vi "Lab Panel V5.29.vi"() -> ()   [LabVIEW 2013] (continued)
                            n1772 = local write "mail control"("END") -> ()
                            n1773 = Bundle(cluster=w3324) -> (w3325:T4)  [unwired: 3 in]
                            n1774 = local write "RUN LAB05-2"(w3322) -> ()
                            n1775 = local write "O/I  LAB05-2"(w3322) -> ()
                            n1776 = local write "run lab05-2"(w3322) -> ()
                            n1777 = local write "DISP LAB05-2"(w3325) -> ()
                          }
                          frame #1 {
                            n1778 = TDMS Close(11:w3326) -> (0:w3327:errorcluster)  [unwired: 1 in, 1 out]
                            n1779 = local write "data file error"(w3327) -> ()
                          }
                          frame #2 {
                            n1780 = stacked-sequence {
                              tunnel: "LAB05-2" -> [w3335 w3341]
                              tunnel: w3332 -> [_ w3340]
                              tunnel: w3331 -> [_ w3339]
                              tunnel: w3330 -> [_ w3338]
                              tunnel: w3329 -> [_ w3337]
                              tunnel: w3328 -> [_ w3336]
                              frame #0 {
                                n1781 = call "sub vi - defrag tdms v1.vi"("panel id"=w3335) -> ("error out"=w3334:errorcluster)  [unwired: 10 in]
                                n1782 = local write "data file error"(w3334) -> ()
                              }
                              frame #1 {
                                n1783 = Bundle("STATUS"=w3340, "OUT SERVER ADDRESS"=w3339, "FROM ACCOUNT"=w3338, "Mail Test File To:"=w3337, "Mail Test Fail"=w3336) -> (w3343:T26)  [unwired: 1 in]
                                n1784 = call "Save data file (pass-fail) v5.vi"("Input Cluster"=w3343, "panel id"=w3341) -> ("network file save error"=w3342:errorcluster)  [unwired: 8 in, 1 out]
                                n1785 = local write "data file error"(w3342) -> ()
                              }
                            }
                          }
                        }
                      }
                    }
                  }
                }
              }
            }
            n1786 = global write "Global display 2.vi" "Mail test file to:"(w2851) -> ()
            n1787 = local read "Network Directory"() -> (w2857:path)
            n1788 = global write "Global 1.vi" "Network Drive"(w2857) -> ()
          }
          frame #8 {
            # "disable functions"
            n1789 = stacked-sequence {
              tunnel: w3353 -> [w3367 _ w3424]
              tunnel: w3352 -> [w3362 _ w3423]
              tunnel: w3351 -> [w3361 _ w3422]
              tunnel: w3350 -> [w3359 _ w3421]
              tunnel: w3349 -> [w3360 _ w3420]
              tunnel: w3348 -> [_ w3384 w3419]
              tunnel: w3347 -> [_ w3385 w3418]
              tunnel: w3346 -> [_ w3386 w3417]
              tunnel: w3345 -> [_ w3387 w3416]
              tunnel: w3344 -> [_ w3388 w3415]
              frame #0 {
                n1790 = Select(t=2, s=w3359, f=0) -> (s? t:f=w3355:i32)
                n1791 = Select(t=2, s=w3361, f=0) -> (s? t:f=w3356:i32)
                n1792 = Select(t=2, s=w3360, f=0) -> (s? t:f=w3354:i32)
                n1793 = Select(t=2, s=w3367, f=0) -> (s? t:f=w3358:i32)
                n1794 = Select(t=2, s=w3362, f=0) -> (s? t:f=w3357:i32)
                n1795 = property on="SELECT LAB02-2" class="RadioBtnsControl (strict)"("DisabledEnum"=w3355) -> ()  [unwired: 2 in, 2 out]
                n1796 = property on="SELECT LAB02-1" class="RadioBtnsControl (strict)"("DisabledEnum"=w3356) -> ()  [unwired: 2 in, 2 out]
                n1797 = property on="SELECT LAB03-1" class="RadioBtnsControl (strict)"("DisabledEnum"=w3354) -> ()  [unwired: 2 in, 2 out]
                n1798 = property on="SELECT LAB01-1" class="RadioBtnsControl (strict)"("DisabledEnum"=w3358) -> ()  [unwired: 2 in, 2 out]
                n1799 = property on="SELECT LAB01-2" class="RadioBtnsControl (strict)"("DisabledEnum"=w3357) -> ()  [unwired: 2 in, 2 out]
                n1800 = Not(x=w3367) -> (.not. x?=w3368:bool)
                n1801 = property on="RESULT LAB01-1" class="Bool (strict)"("Visible"=w3368) -> ()  [unwired: 2 in, 2 out]
                n1802 = Not(x=w3362) -> (.not. x?=w3366:bool)
                n1803 = Not(x=w3361) -> (.not. x?=w3365:bool)
                n1804 = Not(x=w3359) -> (.not. x?=w3364:bool)
                n1805 = property on="RESULT LAB01-2" class="Bool (strict)"("Visible"=w3366) -> ()  [unwired: 2 in, 2 out]
                n1806 = Not(x=w3360) -> (.not. x?=w3363:bool)
                n1807 = property on="RESULT LAB02-1" class="Bool (strict)"("Visible"=w3365) -> ()  [unwired: 2 in, 2 out]
                n1808 = property on="RESULT LAB02-2" class="Bool (strict)"("Visible"=w3364) -> ()  [unwired: 2 in, 2 out]
                n1809 = property on="RESULT LAB03-1" class="Bool (strict)"("Visible"=w3363) -> ()  [unwired: 2 in, 2 out]
                n1810 = property on="SET LAB01-1" class="Clust (strict)"("DisabledEnum"=w3358) -> ()  [unwired: 2 in, 2 out]
                n1811 = property on="SET LAB01-2" class="Clust (strict)"("DisabledEnum"=w3357) -> ()  [unwired: 2 in, 2 out]
                n1812 = property on="SET LAB02-1" class="Clust (strict)"("DisabledEnum"=w3356) -> ()  [unwired: 2 in, 2 out]
                n1813 = property on="SET LAB02-2" class="Clust (strict)"("DisabledEnum"=w3355) -> ()  [unwired: 2 in, 2 out]
                n1814 = property on="SET LAB03-1" class="Clust (strict)"("DisabledEnum"=w3354) -> ()  [unwired: 2 in, 2 out]
                n1815 = property on="O/I  LAB01-1" class="Bool (strict)"("DisabledEnum"=w3358) -> ()  [unwired: 2 in, 2 out]
                n1816 = property on="O/I  LAB01-2" class="Bool (strict)"("DisabledEnum"=w3357) -> ()  [unwired: 2 in, 2 out]
                n1817 = property on="O/I  LAB02-1" class="Bool (strict)"("DisabledEnum"=w3356) -> ()  [unwired: 2 in, 2 out]
                n1818 = property on="O/I  LAB02-2" class="Bool (strict)"("DisabledEnum"=w3355) -> ()  [unwired: 2 in, 2 out]
                n1819 = property on="O/I  LAB03-1" class="Bool (strict)"("DisabledEnum"=w3354) -> ()  [unwired: 2 in, 2 out]
              }
              frame #1 {
                n1820 = Select(t=2, s=w3388, f=0) -> (s? t:f=w3379:i32)
                n1821 = Select(t=2, s=w3387, f=0) -> (s? t:f=w3380:i32)
                n1822 = Select(t=2, s=w3384, f=0) -> (s? t:f=w3383:i32)
                n1823 = Select(t=2, s=w3385, f=0) -> (s? t:f=w3382:i32)
                n1824 = Select(t=2, s=w3386, f=0) -> (s? t:f=w3381:i32)
                n1825 = property on="SELECT LAB05-2" class="RadioBtnsControl (strict)"("DisabledEnum"=w3379) -> ()  [unwired: 2 in, 2 out]
                n1826 = property on="SELECT LAB05-1" class="RadioBtnsControl (strict)"("DisabledEnum"=w3380) -> ()  [unwired: 2 in, 2 out]
                n1827 = property on="SELECT LAB03-2" class="RadioBtnsControl (strict)"("DisabledEnum"=w3383) -> ()  [unwired: 2 in, 2 out]
                n1828 = property on="SELECT LAB04-1" class="RadioBtnsControl (strict)"("DisabledEnum"=w3382) -> ()  [unwired: 2 in, 2 out]
                n1829 = property on="SELECT LAB04-2" class="RadioBtnsControl (strict)"("DisabledEnum"=w3381) -> ()  [unwired: 2 in, 2 out]
                n1830 = property on="SET LAB05-2" class="Clust (strict)"("DisabledEnum"=w3379) -> ()  [unwired: 2 in, 2 out]
                n1831 = property on="SET LAB05-1" class="Clust (strict)"("DisabledEnum"=w3380) -> ()  [unwired: 2 in, 2 out]
                n1832 = property on="SET LAB03-2" class="Clust (strict)"("DisabledEnum"=w3383) -> ()  [unwired: 2 in, 2 out]
                n1833 = property on="SET LAB04-1" class="Clust (strict)"("DisabledEnum"=w3382) -> ()  [unwired: 2 in, 2 out]
                n1834 = property on="SET LAB04-2" class="Clust (strict)"("DisabledEnum"=w3381) -> ()  [unwired: 2 in, 2 out]
                n1835 = property on="O/I  LAB05-2" class="Bool (strict)"("DisabledEnum"=w3379) -> ()  [unwired: 2 in, 2 out]
                n1836 = property on="O/I  LAB05-1" class="Bool (strict)"("DisabledEnum"=w3380) -> ()  [unwired: 2 in, 2 out]
                n1837 = property on="O/I  LAB04-1" class="Bool (strict)"("DisabledEnum"=w3382) -> ()  [unwired: 2 in, 2 out]
                n1838 = property on="O/I  LAB04-2" class="Bool (strict)"("DisabledEnum"=w3381) -> ()  [unwired: 2 in, 2 out]
                n1839 = property on="O/I  LAB03-2" class="Bool (strict)"("DisabledEnum"=w3383) -> ()  [unwired: 2 in, 2 out]
                n1840 = Not(x=w3388) -> (.not. x?=w3389:bool)
                n1841 = Not(x=w3387) -> (.not. x?=w3390:bool)
                n1842 = Not(x=w3386) -> (.not. x?=w3391:bool)
                n1843 = property on="RESULT LAB05-2" class="Bool (strict)"("Visible"=w3389) -> ()  [unwired: 2 in, 2 out]
                n1844 = property on="RESULT LAB05-1" class="Bool (strict)"("Visible"=w3390) -> ()  [unwired: 2 in, 2 out]
                n1845 = Not(x=w3385) -> (.not. x?=w3392:bool)
                n1846 = property on="RESULT LAB04-2" class="Bool (strict)"("Visible"=w3391) -> ()  [unwired: 2 in, 2 out]
                n1847 = Not(x=w3384) -> (.not. x?=w3393:bool)
                n1848 = property on="RESULT LAB04-1" class="Bool (strict)"("Visible"=w3392) -> ()  [unwired: 2 in, 2 out]
                n1849 = property on="RESULT LAB03-2" class="Bool (strict)"("Visible"=w3393) -> ()  [unwired: 2 in, 2 out]
              }
              frame #2 {
                # "disable calibrate if any test running"
                n1850 = Or(x=w3416, y=w3415) -> (x .or. y?=w3409:bool)
                n1851 = Or(x=w3418, y=w3417) -> (x .or. y?=w3411:bool)
                n1852 = Or(x=w3422, y=w3421) -> (x .or. y?=w3413:bool)
                n1853 = Or(x=w3420, y=w3419) -> (x .or. y?=w3412:bool)
                n1854 = Or(x=w3424, y=w3423) -> (x .or. y?=w3414:bool)
                n1855 = Or(x=w3412, y=w3411) -> (x .or. y?=w3410:bool)
                n1856 = Or(x=w3414, y=w3413) -> (x .or. y?=w3408:bool)
                n1857 = Or(x=w3410, y=w3409) -> (x .or. y?=w3407:bool)
                n1858 = Or(x=w3408, y=w3407) -> (x .or. y?=w3404:bool)
                "Any Test Running" <- w3404
                n1859 = case shown="False" w3404 {
                  tunnel: [0 2] -> w3406
                  frame False {
                  }
                  frame True {
                  }
                }
                n1860 = property on="JIG TEST" class="Clust (strict)"("DisabledEnum"=w3406) -> ()  [unwired: 2 in, 2 out]
                n1861 = property on="Network Directory" class="Path"("DisabledEnum"=w3406) -> ()  [unwired: 2 in, 2 out]
                n1862 = property on="MAIL SETTINGS" class="Clust (strict)"("DisabledEnum"=w3406) -> ()  [unwired: 2 in, 2 out]
                n1863 = property on="SET (cal)" class="Bool (strict)"("DisabledEnum"=w3406) -> ()  [unwired: 2 in, 2 out]
                n1864 = property on="ADMIN" class="Bool (strict)"("DisabledEnum"=0) -> ()  [unwired: 2 in, 2 out]
              }
            }
          }
          frame #9 {
            # "drive jigs"
            n1865 = stacked-sequence {
              frame #0 {
                # "jig on"
                n1866 = local read "jig cycle"() -> (w3432:dbl)
                n1867 = property on="JIG TEST" class="Clust (strict)"() -> ("DisabledEnum"=w3429:T16)  [unwired: 2 in, 2 out]
                n1868 = Equal?(x=w3429, y=2) -> (x = y?=w3428:bool)
                n1869 = Equal?(x=w3432, y=0) -> (x = y?=w3430:bool)
                n1870 = And(x=w3430, y=w3428) -> (x .and. y?=w3427:bool)
                n1871 = case shown="True" w3427 {
                  frame False {
                  }
                  frame True {
                    n1872 = local read "run lab01-1"() -> (w3443:bool)
                    n1873 = local read "run lab01-2"() -> (w3442:bool)
                    n1874 = local read "run lab02-1"() -> (w3441:bool)
                    n1875 = local read "run lab02-2"() -> (w3440:bool)
                    n1876 = local read "run lab03-1"() -> (w3439:bool)
                    n1877 = local read "run lab03-2"() -> (w3438:bool)
                    n1878 = local read "run lab04-1"() -> (w3437:bool)
                    n1879 = local read "run lab04-2"() -> (w3436:bool)
                    n1880 = local read "run lab05-1"() -> (w3435:bool)
                    n1881 = local read "run lab05-2"() -> (w3434:bool)
                    n1882 = local write "JIG LAB03-2"(w3438) -> ()
                    n1883 = local write "JIG LAB01-1"(w3443) -> ()
                    n1884 = local write "JIG LAB01-2"(w3442) -> ()
                    n1885 = local write "JIG LAB02-1"(w3441) -> ()
                    n1886 = local write "JIG LAB02-2"(w3440) -> ()
                    n1887 = local write "JIG LAB03-1"(w3439) -> ()
                    n1888 = local write "JIG LAB04-1"(w3437) -> ()
                    n1889 = local write "JIG LAB04-2"(w3436) -> ()
                    n1890 = local write "JIG LAB05-1"(w3435) -> ()
                    n1891 = local write "JIG LAB05-2"(w3434) -> ()
                  }
                }
              }
              frame #1 {
                # "jig off"
                n1892 = local read "jig cycle"() -> (w3450:dbl)
                n1893 = local read "on loops"() -> (w3449:dbl)
                n1894 = property on="JIG TEST" class="Clust (strict)"() -> ("DisabledEnum"=w3448:T16)  [unwired: 2 in, 2 out]
                n1895 = Equal?(x=w3448, y=2) -> (x = y?=w3446:bool)
                n1896 = Equal?(x=w3450, y=w3449) -> (x = y?=w3445:bool)
                n1897 = And(x=w3445, y=w3446) -> (x .and. y?=w3444:bool)
                n1898 = case shown="True" w3444 {
                  frame False {
                  }
                  frame True {
                    w3501 = FALSE
                    w3502 = TRUE
                    w3500 = 2
                    n1899 = local read "SELECT LAB05-2"() -> (w3491:T3)
                    n1900 = local read "SELECT LAB04-2"() -> (w3493:T3)
                    n1901 = local read "SELECT LAB04-1"() -> (w3494:T3)
                    n1902 = local read "SELECT LAB05-1"() -> (w3492:T3)
                    n1903 = local read "SELECT LAB03-2"() -> (w3495:T3)
                    n1904 = local read "SELECT LAB02-1"() -> (w3498:T3)
                    n1905 = local read "SELECT LAB03-1"() -> (w3496:T3)
                    n1906 = local read "SELECT LAB02-2"() -> (w3497:T3)
                    n1907 = local read "SELECT LAB01-2"() -> (w3499:T3)
                    n1908 = local read "run lab05-1"() -> (w3461:bool)
                    n1909 = local read "run lab05-2"() -> (w3460:bool)
                    n1910 = local read "SELECT LAB01-1"() -> (w3503:T3)
                    n1911 = local read "run lab04-2"() -> (w3462:bool)
                    n1912 = local read "run lab04-1"() -> (w3463:bool)
                    n1913 = local read "run lab01-1"() -> (w3479:bool)
                    n1914 = local read "run lab01-2"() -> (w3468:bool)
                    n1915 = local read "run lab03-2"() -> (w3464:bool)
                    n1916 = local read "run lab03-1"() -> (w3465:bool)
                    n1917 = local read "run lab02-1"() -> (w3467:bool)
                    n1918 = local read "run lab02-2"() -> (w3466:bool)
                    n1919 = Equal?(x=w3500, y=w3496) -> (x = y?=w3474:bool)
                    n1920 = Equal?(x=w3500, y=w3495) -> (x = y?=w3473:bool)
                    n1921 = Equal?(x=w3500, y=w3494) -> (x = y?=w3472:bool)
                    n1922 = Equal?(x=w3500, y=w3493) -> (x = y?=w3471:bool)
                    n1923 = Equal?(x=w3500, y=w3492) -> (x = y?=w3470:bool)
                    n1924 = Equal?(x=w3500, y=w3491) -> (x = y?=w3469:bool)
                    n1925 = Equal?(x=w3500, y=w3503) -> (x = y?=w3480:bool)
                    n1926 = Equal?(x=w3500, y=w3498) -> (x = y?=w3476:bool)
                    n1927 = Equal?(x=w3500, y=w3497) -> (x = y?=w3475:bool)
                    n1928 = Equal?(x=w3500, y=w3499) -> (x = y?=w3477:bool)
                    n1929 = And(x=w3471, y=w3462) -> (x .and. y?=w3453:bool)
                    n1930 = And(x=w3474, y=w3465) -> (x .and. y?=w3456:bool)
                    n1931 = And(x=w3472, y=w3463) -> (x .and. y?=w3454:bool)
                    n1932 = And(x=w3469, y=w3460) -> (x .and. y?=w3451:bool)
                    n1933 = And(x=w3475, y=w3466) -> (x .and. y?=w3457:bool)
                    n1934 = And(x=w3473, y=w3464) -> (x .and. y?=w3455:bool)
                    n1935 = And(x=w3470, y=w3461) -> (x .and. y?=w3452:bool)
                    n1936 = And(x=w3477, y=w3468) -> (x .and. y?=w3459:bool)
                    n1937 = And(x=w3480, y=w3479) -> (x .and. y?=w3478:bool)
                    n1938 = And(x=w3476, y=w3467) -> (x .and. y?=w3458:bool)
                    n1939 = Select(t=w3502, s=w3478, f=w3501) -> (s? t:f=w3481:bool)
                    n1940 = Select(t=w3502, s=w3459, f=w3501) -> (s? t:f=w3482:bool)
                    n1941 = Select(t=w3502, s=w3458, f=w3501) -> (s? t:f=w3483:bool)
                    n1942 = Select(t=w3502, s=w3457, f=w3501) -> (s? t:f=w3484:bool)
                    n1943 = Select(t=w3502, s=w3456, f=w3501) -> (s? t:f=w3485:bool)
                    n1944 = Select(t=w3502, s=w3455, f=w3501) -> (s? t:f=w3486:bool)
                    n1945 = Select(t=w3502, s=w3454, f=w3501) -> (s? t:f=w3487:bool)
                    n1946 = Select(t=w3502, s=w3453, f=w3501) -> (s? t:f=w3488:bool)
                    n1947 = Select(t=w3502, s=w3452, f=w3501) -> (s? t:f=w3489:bool)
                    n1948 = Select(t=w3502, s=w3451, f=w3501) -> (s? t:f=w3490:bool)
                    n1949 = local write "JIG LAB03-2"(w3486) -> ()
                    n1950 = local write "JIG LAB02-1"(w3483) -> ()
                    n1951 = local write "JIG LAB02-2"(w3484) -> ()
                    n1952 = local write "JIG LAB01-2"(w3482) -> ()
                    n1953 = local write "JIG LAB03-1"(w3485) -> ()
                    n1954 = local write "JIG LAB01-1"(w3481) -> ()
                    n1955 = local write "JIG LAB05-2"(w3490) -> ()
                    n1956 = local write "JIG LAB04-1"(w3487) -> ()
                    n1957 = local write "JIG LAB05-1"(w3489) -> ()
                    n1958 = local write "JIG LAB04-2"(w3488) -> ()
                  }
                }
              }
            }
          }
          frame #10 {
            # "enable  jig test output if no test busy"
            n1959 = property on="JIG TEST" class="Clust (strict)"() -> ("DisabledEnum"=w3506:T16)  [unwired: 2 in, 2 out]
            n1960 = Equal?(x=w3506, y=0) -> (x = y?=w3504:bool)
            n1961 = case shown="True" w3504 {
              frame False {
              }
              frame True {
                n1962 = local read "JIG TEST"() -> (w3517:T10)
                n1963 = Unbundle(w3517) -> ("LAB01-1"=w3516:bool, "LAB01-2"=w3515:bool, "LAB02-1"=w3514:bool, "LAB02-2"=w3513:bool, "LAB03-1"=w3512:bool, "LAB03-2"=w3511:bool, "LAB04-1"=w3510:bool, "LAB04-2"=w3509:bool, "LAB05-1"=w3508:bool, "LAB05-2"=w3507:bool)
                n1964 = local write "JIG LAB05-1"(w3508) -> ()
                n1965 = local write "JIG LAB05-2"(w3507) -> ()
                n1966 = local write "JIG LAB04-1"(w3510) -> ()
                n1967 = local write "JIG LAB04-2"(w3509) -> ()
                n1968 = local write "JIG LAB03-2"(w3511) -> ()
                n1969 = local write "JIG LAB01-1"(w3516) -> ()
                n1970 = local write "JIG LAB02-1"(w3514) -> ()
                n1971 = local write "JIG LAB03-1"(w3512) -> ()
                n1972 = local write "JIG LAB01-2"(w3515) -> ()
                n1973 = local write "JIG LAB02-2"(w3513) -> ()
              }
            }
          }
          frame #11 {
            w3518 = FALSE
            # "Drive digital output and reset USB and temperature network if required."
            n1974 = global read "Global display 3.vi" "cycle O/F"() -> (w3527:bool)
            n1975 = local read "O/I  LAB05-2"() -> (w3520:bool)
            n1976 = local read "O/I  LAB05-1"() -> (w3522:bool)
            n1977 = local read "JIG LAB05-2"() -> (w3519:bool)
            n1978 = local read "O/I  LAB04-2"() -> (w3524:bool)
            n1979 = local read "JIG LAB05-1"() -> (w3521:bool)
            n1980 = local read "JIG LAB04-2"() -> (w3523:bool)
            n1981 = local read "O/I  LAB03-1"() -> (w3538:bool)
            n1982 = local read "O/I  LAB04-1"() -> (w3534:bool)
            n1983 = local read "O/I  LAB02-1"() -> (w3542:bool)
            n1984 = local read "O/I  LAB02-2"() -> (w3540:bool)
            n1985 = local read "O/I  LAB03-2"() -> (w3536:bool)
            n1986 = local read "JIG LAB04-1"() -> (w3533:bool)
            n1987 = local read "JIG LAB03-2"() -> (w3535:bool)
            n1988 = local read "O/I  LAB01-2"() -> (w3544:bool)
            n1989 = local read "JIG LAB02-1"() -> (w3541:bool)
            n1990 = local read "JIG LAB02-2"() -> (w3539:bool)
            n1991 = local read "JIG LAB03-1"() -> (w3537:bool)
            n1992 = local read "O/I  LAB01-1"() -> (w3546:bool)
            n1993 = local read "JIG LAB01-2"() -> (w3543:bool)
            n1994 = local read "JIG LAB01-1"() -> (w3545:bool)
            n1995 = case shown="False" w3527 {
              tunnel: [w3659 FALSE] -> w3526
              frame False {
                n1996 = local read "Analog error"() -> (w3661:bool)
                n1997 = local read "Reset Measuring"() -> (w3660:bool)
                n1998 = Or(x=w3660, y=w3661) -> (x .or. y?=w3659:bool)
              }
              frame True {
              }
            }
            n1999 = Build Array(w3539, w3538, w3537, w3536, w3535, w3534, w3533) -> (w3531:bool[])
            "USB OUT 1" <- w3531
            n2000 = Build Array(w3546, w3545, w3544, w3543, w3542, w3541, w3540) -> (w3532:bool[])
            "USB OUT 0" <- w3532
            n2001 = Build Array(w3524, w3523, w3522, w3521, w3520, w3519, w3518, w3518) -> (w3530:bool[])
            "USB OUT 2" <- w3530
            n2002 = Not(x=w3527) -> (.not. x?=w3528:bool)
            n2003 = local read "Simulate"() -> (w3529:bool)
            n2004 = And(x=w3528, y=w3526) -> (x .and. y?=w3525:bool)
            n2005 = stacked-sequence {
              tunnel: w3532 -> [w3550 w3556]
              tunnel: w3531 -> [w3549 w3555]
              tunnel: w3530 -> [w3548 w3554]
              tunnel: w3529 -> [w3547 w3557]
              tunnel: w3525 -> [_ w3558]
              frame #0 {
                # "drive outputs for normal use"
                n2006 = case shown="False" w3547 {
                  tunnel: w3550 -> [w3553 _]
                  tunnel: w3549 -> [w3552 _]
                  tunnel: w3548 -> [w3551 _]
                  frame False {
                    n2007 = call "sub vi - Drive Relays All v6.vi"("Array #2"=w3551, "Array #1"=w3552, "Array #0"=w3553) -> ()  [unwired: 8 in, 1 out]
                  }
                  frame True {
                  }
                }
              }
              frame #1 {
                # "USB  reset routine"
                n2008 = case shown="True" w3558 {
                  tunnel: w3557 -> [_ w3562]
                  tunnel: w3556 -> [_ w3561]
                  tunnel: w3555 -> [_ w3560]
                  tunnel: w3554 -> [_ w3559]
                  frame False {
                  }
                  frame True {
                    n2009 = stacked-sequence {
                      seq-local: [w3564 _ _ _ _] -> [_ w3570 _ _ _]
                      tunnel: w3562 -> [_ w3574 _ _ _]
                      tunnel: w3561 -> [_ w3573 _ _ _]
                      tunnel: w3560 -> [_ w3572 _ _ _]
                      tunnel: w3559 -> [_ w3571 _ _ _]
                      frame #0 {
                        n2010 = case shown="False" "Auto Reset" {
                          tunnel: [w3567 FALSE] -> w3565
                          frame False {
                            n2011 = Two Button Dialog(message="System reset") -> (T button?=w3567:bool)  [unwired: 2 in]
                          }
                          frame True {
                          }
                        }
                        n2012 = disable-structure shown="Disabled" {
                          frame Disabled {
                            n2013 = local write "Tab Control 2"(5) -> ()
                          }
                          frame Enabled {
                          }
                        }
                        n2014 = Or(x="Auto Reset", y=w3565) -> (x .or. y?=w3564:bool)
                      }
                      frame #1 {
                        n2015 = case shown="True" w3570 {
                          tunnel: w3574 -> [_ w3580]
                          tunnel: w3573 -> [_ w3579]
                          tunnel: w3572 -> [_ w3578]
                          tunnel: w3571 -> [_ w3577]
                          frame False {
                          }
                          frame True {
                            n2016 = stacked-sequence {
                              tunnel: w3580 -> [_ w3598 _]
                              tunnel: bool[] [] -> [w3583 w3597 w3616]
                              tunnel: w3579 -> [_ _ w3615]
                              tunnel: w3578 -> [w3582 _ w3614]
                              tunnel: w3577 -> [w3581 _ w3613]
                              tunnel: 5000 -> [w3584 _ w3612]
                              frame #0 {
                                # "switch off test stations for system reset"
                                n2017 = stacked-sequence {
                                tunnel: w3584 -> [w3588 w3592 w3594]
                                tunnel: w3583 -> [w3587 w3591 w3595]
                                tunnel: w3582 -> [w3586 _ _]
                                tunnel: w3581 -> [w3585 w3590 _]
                                frame #0 {
                                # "drive 1st 7 inputs"
                                n2018 = call "sub vi - Drive Relays All v6.vi"("Array #2"=w3585, "Array #1"=w3586, "Array #0"=w3587) -> ()  [unwired: 8 in, 1 out]
                                n2019 = call "Message Display V1.vi"("Message"="Delay off LAB 01-1 to 02-1", "Delay mS"=w3588) -> ()  [unwired: 10 in]
                                }
                                frame #1 {
                                # "drive 2nd 7 inputs"
                                n2020 = call "sub vi - Drive Relays All v6.vi"("Array #2"=w3590, "Array #1"=w3591, "Array #0"=w3591) -> ()  [unwired: 8 in, 1 out]
                                n2021 = call "Message Display V1.vi"("Message"="Delay off LAB 02-2 to 04-1", "Delay mS"=w3592) -> ()  [unwired: 10 in]
                                }
                                frame #2 {
                                # "drive 3rd 7 inputs"
                                n2022 = call "sub vi - Drive Relays All v6.vi"("Array #2"=w3595, "Array #1"=w3595, "Array #0"=w3595) -> ()  [unwired: 8 in, 1 out]
                                n2023 = call "Message Display V1.vi"("Message"="Delay off LAB 04-2 to 05-2", "Delay mS"=w3594) -> ()  [unwired: 10 in]
                                }
                                }
                              }
                              frame #1 {
                                # "reset all usb modules"
                                n2024 = stacked-sequence {
                                tunnel: w3598 -> [_ w3603]
                                tunnel: w3597 -> [w3601 _]
                                frame #0 {
                                n2025 = local write "AI Task"(FALSE) -> ()
                                n2026 = call "sub vi - Drive Relays All v6.vi"("Array #2"=bool[] [FALSE, FALSE, FALSE, FALSE, FALSE, FALSE, TRUE, FALSE], "Array #1"=w3601, "Array #0"=w3601) -> ()  [unwired: 8 in, 1 out]
                                }
                                frame #1 {
                                n2027 = call "Reset Meas v 5.vi"("simulate"=w3603) -> ("Reset Error"=w3602:bool)  [unwired: 10 in]
                                n2028 = case shown="False" w3602 {
                                frame False {
                                n2029 = local read "RATE (Hz)"() -> (w3607:dbl)
                                n2030 = local read "SAMPLES"() -> (w3606:dbl)
                                n2031 = call "sub vi - AI USB4704 (3)  Create Task v4.vi"("Rate Hz"=w3607, "Samples"=w3606) -> ("TASK USB 0"=w3610:i32, "TASK USB 1"=w3609:i32, "TASK USB 2"=w3608:i32, "AI Task Er"=w3604:bool)  [unwired: 9 in, 1 out]
                                n2032 = local write "AI Task"(TRUE) -> ()
                                n2033 = local write "Reset Error"(w3604) -> ()
                                n2034 = local write "AI Task2"(w3608) -> ()
                                n2035 = local write "AI Task1"(w3609) -> ()
                                n2036 = local write "AI Task0"(w3610) -> ()
                                }
                                frame True {
                                "Reset Error" <- TRUE
                                }
                                }
                                }
                                }
                              }
                              frame #2 {
                                # "switch test stations back on after reset"
                                n2037 = stacked-sequence {
                                tunnel: w3616 -> [w3620 w3623 _]
                                tunnel: w3615 -> [w3619 w3625 w3630]
                                tunnel: w3612 -> [w3618 w3621 w3627]
                                tunnel: w3614 -> [_ w3624 w3629]
                                tunnel: w3613 -> [_ _ w3626]
                                frame #0 {
                                # "drive 1st 7 inputs"
                                n2038 = call "sub vi - Drive Relays All v6.vi"("Array #2"=w3620, "Array #1"=w3620, "Array #0"=w3619) -> ()  [unwired: 8 in, 1 out]
                                n2039 = call "Message Display V1.vi"("Message"="Delay on LAB 01-1 to 02-1", "Delay mS"=w3618) -> ()  [unwired: 10 in]
                                }
                                frame #1 {
                                # "drive 1st & 2nd outputs"
                                n2040 = call "sub vi - Drive Relays All v6.vi"("Array #2"=w3623, "Array #1"=w3624, "Array #0"=w3625) -> ()  [unwired: 8 in, 1 out]
                                n2041 = call "Message Display V1.vi"("Message"="Delay on LAB 02-2 to 04-1", "Delay mS"=w3621) -> ()  [unwired: 10 in]
                                }
                                frame #2 {
                                n2042 = call "sub vi - Drive Relays All v6.vi"("Array #2"=w3626, "Array #1"=w3629, "Array #0"=w3630) -> ()  [unwired: 8 in, 1 out]
                                n2043 = call "Message Display V1.vi"("Message"="Delay on LAB 04-2 to 05-2", "Delay mS"=w3627) -> ()  [unwired: 10 in]
                                }
                                }
                              }
                            }
                          }
                        }
                      }
                      frame #2 {
                        w3631 = 0
                        w3632 = FALSE
                        # "set all back to zero"
                        n2044 = local read "Total USB resets"() -> (w3634:dbl)
                        n2045 = local read "Resets Done"() -> (w3636:dbl)
                        n2046 = local write "Reset Measuring"(w3632) -> ()
                        n2047 = local write "Analog error"(w3632) -> ()
                        n2048 = local write "Er USB#2"(w3631) -> ()
                        n2049 = local write "Er USB#0"(w3631) -> ()
                        n2050 = local write "Er USB#1"(w3631) -> ()
                        n2051 = local write "Error USB #0"(w3632) -> ()
                        n2052 = local write "Error USB #1"(w3632) -> ()
                        n2053 = local write "Error USB #2"(w3632) -> ()
                        n2054 = Increment(x=w3634) -> (x+1=w3633:dbl)
                        n2055 = Increment(x=w3636) -> (x+1=→"Resets Done":dbl)
                        n2056 = local write "Total USB resets"(w3633) -> ()
                      }
                      frame #3 {
                        # "save reset value"
                        n2057 = String To Path(string="c:\\crabtree\\Set Up\\") -> (path=w3646:path)
                        n2058 = Build Path(base path=w3646, name or relative path="USB resets.bin") -> (appended path=w3639:path)
                        n2059 = Create Folder(path (use dialog)=w3646) -> (error out=w3638:errorcluster)  [unwired: 2 in, 2 out]
                        n2060 = local read "Total USB resets"() -> (w3637:dbl)
                        n2061 = call <vilib>:"Clear Errors.vi"("error in (no error)"=w3638) -> ()  [unwired: 6 in, 1 out]
                        n2062 = Open/Create/Replace File(file path (use dialog)=w3639, operation (0:open)=T17."replace or create") -> (refnum out=w3644:refnum<file>, error out=w3643:errorcluster)  [unwired: 4 in, 1 out]
                        n2063 = Write to Binary File(file (use dialog)=w3644, data=w3637, error in=w3643) -> (refnum out=w3642:refnum<file>, error out=w3641:errorcluster)  [unwired: 3 in, 1 out]
                        n2064 = Close File(refnum=w3642, error in=w3641) -> (error out=w3640:errorcluster)  [unwired: 1 out]
                        n2065 = local write "data file error"(w3640) -> ()
                      }
                      frame #4 {
                        # "mail reset value"
                        n2066 = local read "MAIL SETTINGS"() -> (w3652:T7)
                        n2067 = local read "Total USB resets"() -> (w3656:dbl)
                        n2068 = Unbundle(w3652) -> ("OUT SERVER ADDRESS"=w3658:string, "FROM ACCOUNT"=w3657:string)  [unwired: 5 out]
                        n2069 = Number To Decimal String(number=w3656) -> (decimal integer string=w3654:string)  [unwired: 1 in]
                        n2070 = Concatenate Strings("Total USB resets: ", w3654) -> (w3653:string)
                        n2071 = call "sub vi - send mail v5.vi"("TO:"="francois@ffg.net", "subject"=w3653, "from"=w3657, "out going server"=w3658) -> ("error out"=w3651:errorcluster)  [unwired: 11 in]
                        n2072 = Bundle(cluster=w3652, "mail error"=w3651) -> (w3650:T7)  [unwired: 6 in]
                        n2073 = local write "MAIL SETTINGS"(w3650) -> ()
                      }
                    }
                  }
                }
              }
            }
          }
          frame #12 {
            # "if all test panels are off stop analog read"
            n2074 = local read "O/I  LAB03-1"() -> (w3684:bool)
            n2075 = local read "O/I  LAB03-2"() -> (w3683:bool)
            n2076 = local read "O/I  LAB04-1"() -> (w3682:bool)
            n2077 = local read "O/I  LAB04-2"() -> (w3681:bool)
            n2078 = local read "O/I  LAB05-1"() -> (w3680:bool)
            n2079 = local read "O/I  LAB05-2"() -> (w3679:bool)
            n2080 = local read "O/I  LAB02-2"() -> (w3685:bool)
            n2081 = local read "O/I  LAB02-1"() -> (w3686:bool)
            n2082 = local read "O/I  LAB01-2"() -> (w3687:bool)
            n2083 = local read "O/I  LAB01-1"() -> (w3688:bool)
            n2084 = Or(x=w3680, y=w3679) -> (x .or. y?=w3677:bool)
            n2085 = Or(x=w3682, y=w3681) -> (x .or. y?=w3678:bool)
            n2086 = Or(x=w3686, y=w3685) -> (x .or. y?=w3676:bool)
            n2087 = Or(x=w3684, y=w3683) -> (x .or. y?=w3674:bool)
            n2088 = Or(x=w3688, y=w3687) -> (x .or. y?=w3675:bool)
            n2089 = Or(x=w3678, y=w3677) -> (x .or. y?=w3671:bool)
            n2090 = Or(x=w3675, y=w3676) -> (x .or. y?=w3673:bool)
            n2091 = Or(x=w3673, y=w3674) -> (x .or. y?=w3672:bool)
            n2092 = local read "Any Test Running"() -> (w3670:bool)
            n2093 = Or(x=w3672, y=w3671) -> (x .or. y?=w3669:bool)
            n2094 = local read "AI Task"() -> (w3665:bool)
            n2095 = Or(x=w3669, y=w3670) -> (x .or. y?=w3664:bool)
            n2096 = Not(x=w3664) -> (.not. x?=w3668:bool)
            n2097 = Not(x=w3665) -> (.not. x?=w3666:bool)
            n2098 = And(x=w3668, y=w3665) -> (x .and. y?=w3667:bool)
            n2099 = And(x=w3664, y=w3666) -> (x .and. y?=w3663:bool)
            n2100 = case shown="True" w3667 {
              frame False {
              }
              frame True {
                # "close task if no test"
                n2101 = local write "AI Task"(FALSE) -> ()
                n2102 = call "sub vi - AI USB4704 (3)  Close Task v2.vi"() -> ()  [unwired: 16 in]
              }
            }
            n2103 = case shown="True" w3663 {
              frame False {
              }
              frame True {
                # "create task for test"
                n2104 = local read "SAMPLES"() -> (w3690:dbl)
                n2105 = local read "RATE (Hz)"() -> (w3689:dbl)
                n2106 = call "sub vi - AI USB4704 (3)  Create Task v4.vi"("Rate Hz"=w3689, "Samples"=w3690) -> ("TASK USB 0"=w3691:i32, "TASK USB 1"=w3692:i32, "TASK USB 2"=w3693:i32)  [unwired: 9 in, 2 out]
                n2107 = local write "AI Task0"(w3691) -> ()
                n2108 = local write "AI Task1"(w3692) -> ()
                n2109 = local write "AI Task2"(w3693) -> ()
                n2110 = local write "AI Task"(TRUE) -> ()
              }
            }
          }
          frame #13 {
            # "get all analog values from USB devices"
            n2111 = local read "on loops"() -> (w3703:dbl)
            n2112 = local read "jig cycle"() -> (w3700:dbl)
            n2113 = Add(x=w3703, y=3) -> (x+y=w3701:dbl)
            n2114 = Equal?(x=w3700, y=3) -> (x = y?=w3698:bool)
            n2115 = Equal?(x=w3700, y=w3701) -> (x = y?=w3699:bool)
            n2116 = Or(x=w3698, y=w3699) -> (x .or. y?=w3697:bool)
            n2117 = global write "Global display 3.vi" "cycle O/F"(w3698) -> ()
            n2118 = case shown="True" w3697 {
              tunnel: w3698 -> [_ w3709]
              tunnel: w3696 -> [_ w3706]
              frame False {
              }
              frame True {
                n2119 = local read "Simulate"() -> (w3712:bool)
                n2120 = case shown="False" w3712 {
                  tunnel: [w3728 dynamicdata[] [] ("array GRAPH")] -> w3718
                  tunnel: [w3727 w3753] -> w3717
                  tunnel: [w3726 w3753] -> w3716
                  tunnel: [w3725 w3753] -> w3715
                  tunnel: [w3724 w3753] -> w3714
                  tunnel: [w3723 w3753] -> w3713
                  tunnel: w3709 -> [_ w3757]
                  tunnel: [w3722 "Ambient Volts"] -> w3708
                  tunnel: [w3721 bool[] []] -> w3707
                  tunnel: w3706 -> [w3720 _]
                  tunnel: [w3719 0.3 ("Analog loop time")] -> w3705
                  frame False {
                    # "analog in"
                    n2121 = case shown="True" w3720 {
                      tunnel: [dynamicdata[] [] ("array GRAPH") w3747] -> w3728
                      tunnel: [w3730 w3746] -> w3727
                      tunnel: [w3730 w3745] -> w3726
                      tunnel: [w3730 w3744] -> w3725
                      tunnel: [w3730 w3743] -> w3724
                      tunnel: [w3730 w3742] -> w3723
                      tunnel: [3 w3741] -> w3722
                      tunnel: [bool[] [] w3740] -> w3721
                      tunnel: [0.0 w3736] -> w3719
                      frame False {
                        w3731 = 0.0
                        # "no test"
                        n2122 = Bundle(w3731, w3731, w3731, w3731, w3731, w3731) -> (w3730:cluster{dbl, dbl, dbl, dbl, dbl, dbl})  [unwired: 1 in]
                      }
                      frame True {
                        # "test on"
                        n2123 = local read "AI data 0"() -> (w3739:waveform(dbl)[])
                        n2124 = local read "AI data 1"() -> (w3738:waveform(dbl)[])
                        n2125 = local read "AI data 2"() -> (w3735:waveform(dbl)[])
                        n2126 = local read "AI Error"() -> (w3737:errorcluster[])
                        n2127 = call "sub vi - Read Analog All v9.5.vi"("data 0"=w3739, "data 1"=w3738, "data 2"=w3735, "AI Error"=w3737) -> ("array GRAPH"=w3747:dynamicdata[], "LAB01"=w3746:T27, "LAB02"=w3745:T28, "LAB03"=w3744:T29, "LAB04"=w3743:T30, "deg C"=w3741:dbl, "USB Error"=w3740:bool[], "LAB05"=w3742:T31)  [unwired: 4 in]
                        n2128 = local read "AI loop time"() -> (w3736:dbl)
                      }
                    }
                  }
                  frame True {
                    # "simulate"
                    n2129 = local read "ON amps"() -> (w3751:dbl)
                    n2130 = local read "OFF amps"() -> (w3752:dbl)
                    n2131 = local read "VOLTS"() -> (w3755:dbl)
                    n2132 = local read "PF"() -> (w3754:dbl)
                    n2133 = Select(t=w3751, s=w3757, f=w3752) -> (s? t:f=w3756:dbl)
                    n2134 = Bundle("OFF amps"=w3756, "VOLTS"=w3755, "PF"=w3754, "OFF amps"=w3756, "VOLTS"=w3755, "PF"=w3754) -> (w3753:T32)  [unwired: 1 in]
                  }
                }
                n2135 = local read "Simulate"() -> (w3711:bool)
                n2136 = stacked-sequence {
                  seq-local: [w3761 _ _ _ _ _ _ _] -> [_ _ _ _ _ _ _ _]
                  seq-local: [w3760 _ _ _ _ _ _ _] -> [_ _ _ _ _ _ _ _]
                  seq-local: [w3759 _ _ _ _ _ _ _] -> [_ _ _ _ _ _ _ w3954]
                  tunnel: w3718 -> [_ w3812 _ _ _ _ _ _]
                  tunnel: w3717 -> [_ _ w3839 _ _ _ _ _]
                  tunnel: w3716 -> [_ _ _ w3867 _ _ _ _]
                  tunnel: w3715 -> [_ _ _ _ w3895 _ _ _]
                  tunnel: w3714 -> [_ _ _ _ _ w3923 _ _]
                  tunnel: w3713 -> [_ _ _ _ _ _ w3951 _]
                  tunnel: w3711 -> [_ _ w3838 w3866 w3894 w3922 w3950 w3956]
                  tunnel: T14 {"1  (A) cal"=1.0, "1 (V) cal"=1.0, "1 (PF) cal"=1.0, "1 (TL) cal"=1.0, "1 (TN) cal"=1.0, "2 (A) cal"=1.0, "2 (V) cal"=1.0, "2 (PF) cal"=1.0, "2 (TL) cal"=1.0, "2 (TN) cal"=1.0} ("CAL LAB01") -> [_ _ w3837 w3865 w3893 w3921 w3949 _]
                  tunnel: w3708 -> [_ _ _ _ _ _ _ w3955]
                  tunnel: w3707 -> [w3764 _ _ _ _ _ _ _]
                  tunnel: w3705 -> [_ w3791 _ _ _ _ _ _]
                  frame #0 {
                    n2137 = Index Array(array=w3764, index=2) -> (element=w3759:bool)
                    n2138 = Index Array(array=w3764, index=1) -> (element=w3760:bool)
                    n2139 = Index Array(array=w3764, index=0) -> (element=w3761:bool)
                    n2140 = local write "Error USB #2"(w3759) -> ()
                    n2141 = local write "Error USB #0"(w3761) -> ()
                    n2142 = local write "Error USB #1"(w3760) -> ()
                    n2143 = stacked-sequence {
                      tunnel: w3761 -> [w3768 _ _ _]
                      tunnel: w3760 -> [_ w3773 _ _]
                      tunnel: 0 -> [w3767 w3772 w3777 _]
                      tunnel: w3759 -> [_ _ w3778 _]
                      frame #0 {
                        n2144 = case shown="True" w3768 {
                          tunnel: w3767 -> [w3769 _]
                          frame False {
                            n2145 = local write "Er USB#0"(w3769) -> ()
                          }
                          frame True {
                            n2146 = local read "Er USB#0"() -> (w3771:dbl)
                            n2147 = Increment(x=w3771) -> (x+1=→"Er USB#0":dbl)
                          }
                        }
                      }
                      frame #1 {
                        n2148 = case shown="True" w3773 {
                          tunnel: w3772 -> [w3774 _]
                          frame False {
                            n2149 = local write "Er USB#1"(w3774) -> ()
                          }
                          frame True {
                            n2150 = local read "Er USB#1"() -> (w3776:dbl)
                            n2151 = Increment(x=w3776) -> (x+1=→"Er USB#1":dbl)
                          }
                        }
                      }
                      frame #2 {
                        n2152 = case shown="True" w3778 {
                          tunnel: w3777 -> [w3779 _]
                          frame False {
                            n2153 = local write "Er USB#2"(w3779) -> ()
                          }
                          frame True {
                            n2154 = local read "Er USB#2"() -> (w3781:dbl)
                            n2155 = Increment(x=w3781) -> (x+1=→"Er USB#2":dbl)
                          }
                        }
                      }
                      frame #3 {
                        w3787 = 10
                        n2156 = local read "Er USB#2"() -> (w3788:dbl)
                        n2157 = local read "Er USB#0"() -> (w3790:dbl)
                        n2158 = local read "Er USB#1"() -> (w3789:dbl)
                        n2159 = Greater Or Equal?(x=w3790, y=w3787) -> (x >= y?=w3785:bool)
                        n2160 = Greater Or Equal?(x=w3789, y=w3787) -> (x >= y?=w3784:bool)
                        n2161 = Greater Or Equal?(x=w3788, y=w3787) -> (x >= y?=w3783:bool)
                        n2162 = Or(x=w3785, y=w3784) -> (x .or. y?=w3786:bool)
                        n2163 = Or(x=w3786, y=w3783) -> (x .or. y?=→"Analog error":bool)
                      }
                    }
                  }
                  frame #1 {
                    # "display graph data on ADM page"
                    n2164 = local write "AI loop time"(w3791) -> ()
                    n2165 = local write "AI"(TRUE) -> ()
                    n2166 = Index Array(array=w3812, index=6) -> (element=→"LAB04-1 (GRAPH)":dynamicdata)
                    n2167 = Index Array(array=w3812, index=7) -> (element=→"LAB04-2 (GRAPH)":dynamicdata)
                    n2168 = Index Array(array=w3812, index=9) -> (element=→"LAB05-2 (GRAPH)":dynamicdata)
                    n2169 = Index Array(array=w3812, index=8) -> (element=→"LAB05-1 (GRAPH)":dynamicdata)
                    n2170 = Index Array(array=w3812, index=5) -> (element=→"LAB03-2 (GRAPH)":dynamicdata)
                    n2171 = Index Array(array=w3812, index=0) -> (element=→"LAB01-1 (GRAPH)":dynamicdata)
                    n2172 = Index Array(array=w3812, index=1) -> (element=→"LAB01-2 (GRAPH)":dynamicdata)
                    n2173 = Index Array(array=w3812, index=2) -> (element=→"LAB02-1 (GRAPH)":dynamicdata)
                    n2174 = Index Array(array=w3812, index=3) -> (element=→"LAB02-2 (GRAPH)":dynamicdata)
                    n2175 = Index Array(array=w3812, index=4) -> (element=→"LAB03-1 (GRAPH)":dynamicdata)
                  }
                  frame #2 {
                    n2176 = case shown="False" w3838 {
                      tunnel: [w3840 w3841] -> w3836
                      tunnel: w3837 -> [_ w3841]
                      frame False {
                        n2177 = local read "CAL LAB01"() -> (w3840:T14)
                      }
                      frame True {
                      }
                    }
                    n2178 = Unbundle By Name(w3839) -> ("OFF amps"=w3835:dbl, "VOLTS"=w3834:dbl, "PF"=w3833:dbl, "OFF amps"=w3832:dbl, "VOLTS"=w3831:dbl, "PF"=w3830:dbl)
                    n2179 = Unbundle By Name(w3836) -> ("1  (A) cal"=w3829:dbl, "1 (V) cal"=w3828:dbl, "1 (PF) cal"=w3827:dbl, "2 (A) cal"=w3826:dbl, "2 (V) cal"=w3825:dbl, "2 (PF) cal"=w3824:dbl)  [unwired: 4 out]
                    n2180 = Multiply(x=w3835, y=w3829) -> (x*y=w3822:dbl)
                    n2181 = Multiply(x=w3834, y=w3828) -> (x*y=w3821:dbl)
                    n2182 = Multiply(x=w3833, y=w3827) -> (x*y=w3820:dbl)
                    n2183 = Multiply(x=w3832, y=w3826) -> (x*y=w3818:dbl)
                    n2184 = Multiply(x=w3831, y=w3825) -> (x*y=w3817:dbl)
                    n2185 = Multiply(x=w3830, y=w3824) -> (x*y=w3816:dbl)
                    n2186 = local read "SIG LAB01-1"() -> (w3823:T2)
                    n2187 = local read "SIG LAB01-2"() -> (w3819:T2)
                    n2188 = Bundle By Name(cluster=w3823, "AMPS"=w3822, "VOLTS"=w3821, "PF"=w3820) -> (w3815:T2)
                    n2189 = Bundle By Name(cluster=w3819, "AMPS"=w3818, "VOLTS"=w3817, "PF"=w3816) -> (w3814:T2)
                    n2190 = global write "Global display 1.vi" "SIG LAB01-2"(w3814) -> ()
                    n2191 = global write "Global display 1.vi" "SIG LAB01-1"(w3815) -> ()
                    n2192 = local write "SIG LAB01-2"(w3814) -> ()
                    n2193 = local write "SIG LAB01-1"(w3815) -> ()
                  }
                  frame #3 {
                    n2194 = Unbundle By Name(w3867) -> ("OFF amps"=w3863:dbl, "VOLTS"=w3862:dbl, "PF"=w3861:dbl, "OFF amps"=w3860:dbl, "VOLTS"=w3859:dbl, "PF"=w3858:dbl)
                    n2195 = case shown="True" w3866 {
                      tunnel: [w3868 w3869] -> w3864
                      tunnel: w3865 -> [_ w3869]
                      frame False {
                        n2196 = local read "CAL LAB02"() -> (w3868:T15)
                      }
                      frame True {
                      }
                    }
                    n2197 = Unbundle By Name(w3864) -> ("1  (A) cal"=w3857:dbl, "1 (V) cal"=w3856:dbl, "1 (PF) cal"=w3855:dbl, "2 (A) cal"=w3854:dbl, "2 (V) cal"=w3853:dbl, "2 (PF) cal"=w3852:dbl)  [unwired: 4 out]
